vi "VI Server_Get Cluster Controls Refferences Without Merging.vi"(7 "Cluster.Label":string, 8 "error in":errorcluster, 11 "VI Server Cluster":T1={"Labels"=["Label", "Size", "Font", "Heght", "Width", "Ledding Denominator", "Ledding Nominator", "Label Number", "Microstep Resolution", "X", "Y", "Z", "Italic?", "Underlined?"], "Refs"=[], "VI Ref"=refnum}) -> (0 "error out":errorcluster, 2 "Cluster.VI Server Cluster":T1={"Labels"=["Label", "Size", "Font", "Heght", "Width", "Ledding Denominator", "Ledding Nominator", "Label Number", "Microstep Resolution", "X", "Y", "Z", "Italic?", "Underlined?"], "Refs"=[], "VI Ref"=refnum}, 3 "VI Server Cluster.DUP":T1={"Labels"=["Label", "Size", "Font", "Heght", "Width", "Ledding Denominator", "Ledding Nominator", "Label Number", "Microstep Resolution", "X", "Y", "Z", "Italic?", "Underlined?"], "Refs"=[], "VI Ref"=refnum})   [LabVIEW 2020, in "VI Server Toolkit LV2013.lvlib"]
doc: "Retrieves cluster's content labels and associated references and outputs them as separate VI Server Cluster.\nThese controls can be accessed via VI Server Tools.\nPlease keep in mind the labels should be unique in order to be properly identified."
uses:
  VI Server Toolkit LV2013.lvlib
  VI Server_TypeDefs/VI Server_RefsCluster.ctl
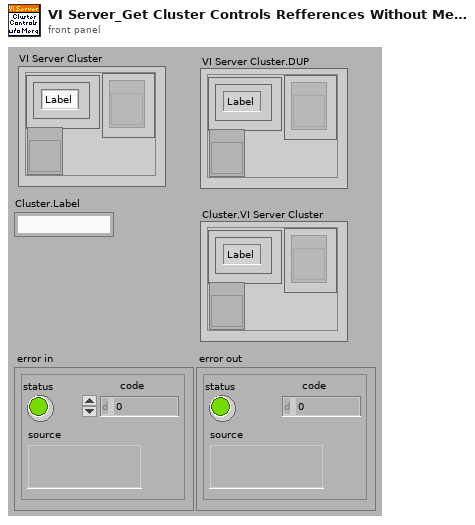
[diagram p1: front panel]
types:
  T1 = typedef "VI Server_RefsCluster.ctl" = cluster{"Labels":string[], "Refs":refnum<vi>[], "VI Ref":refnum<vi>}
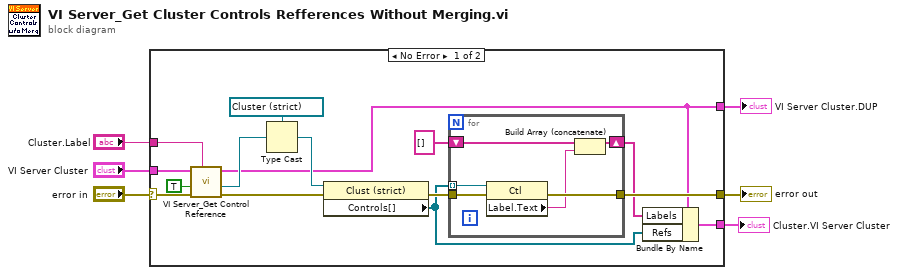
[diagram p0: block diagram]
diagram:
  n1 = case shown="No Error" "error in" {
    selector: "error in" -> [w18 w29]
    tunnel: "VI Server Cluster" -> [w16 _]
    tunnel: [w21 w29] -> w5
    tunnel: [w10 w28] -> w3
    tunnel: "Cluster.Label" -> [w15 _]
    tunnel: [w7 _] -> w1
    frame No Error {
      n2 = call "VI Server_Get Control Reference.vi"("Label"=w15, "error in"=w18, "Single Instance (T)"=TRUE, "VI Server Cluster"=w16) -> ("error out"=w17:errorcluster, "Control Reference (Generic)"=w14:refnum<vi>, "VI Server Cluster.DUP"=w10:T1)  [unwired: 4 in, 1 out]
      n3 = Type Cast(type=refnum<vi> refnum ("VI ServerCluster"), x=w14) -> (*(type *) &x=w13:refnum<vi>)
      n4 = property class="Clust (strict)"(reference=w13, error in=w17) -> (error out=w20:errorcluster, "Controls[]"=w8:refnum<vi>[])  [unwired: 1 out]
      n5 = for {
        tunnel: w20 -> [w22]
        tunnel: [w27] -> w21
        tunnel: w8 -> [w23] mode=indexing
        shift-right: [w24] -> w9
        shift-left: string[] [] -> [w26]
        n6 = property class="Ctl"(reference=w23, error in=w22) -> (error out=w27:errorcluster, "Label.Text"=w25:string)  [unwired: 1 out]
        n7 = Build Array (concatenate)(w26, w25) -> (w24:string[])
      }
      n8 = Bundle By Name(cluster=w10, "Labels"=w9, "Refs"=w8) -> (w7:T1)
    }
    frame Error {
      n9 = call "VI Server_Empty VI Server Cluster.vi"() -> ("VI Server Cluster"=w28:T1)  [unwired: 7 in]
    }
  }
  "error out" <- w5
  "VI Server Cluster.DUP" <- w3
  "Cluster.VI Server Cluster" <- w1
